vi "Module Name--constant.vi"() -> (3 "Module Name":string)   [LabVIEW 2019, in "ContextHelp.lvlib"]
doc: "Return the name of the module that owns this VI. \n_____\nBased on DQMH Project Template 6.1.0.94.\n____\nPantherLAB Templates 1.0.0.5\nCopyright (c) 2022, PantherLAB"
uses:
  ContextHelp.lvlib
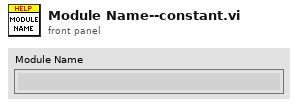
[diagram p1: front panel]
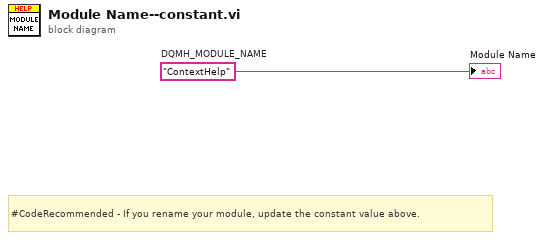
[diagram p0: block diagram]
diagram:
  w1 = "ContextHelp"  # DQMH_MODULE_NAME
  # "#CodeRecommended - If you rename your module, update the constant value above."
  "Module Name" <- w1
